vi "main.vi"() -> ()   [LabVIEW 2015]
uses:
  USB Template (LV 8.6)/Boiler/Controls/Boiler Controls.ctl
  USB Template (LV 8.6)/Boiler/Controls/Boiler Simulation Controls.ctl
  USB Template (LV 8.6)/Boiler/Controls/Boiler Status Indicators.ctl
  status.ctl
  boiler data.ctl
  log info.ctl
  timerstatus.ctl
panel:
  out "error out":errorcluster
  in  "stop":bool
  out "Boiler Status Indicators":T1 {"Time Count" format="%.2g"}
  in  "Boiler Simulation Controls":T2 {"Flame Sensor Value (%)" min=0.0 max=100.0 scale=0.0..100.0}
  in  "Boiler Controls":T3 {"Fuel Valve Position" min=0.0 max=100.0 scale=0.0..100.0 scale format="%.2f"}
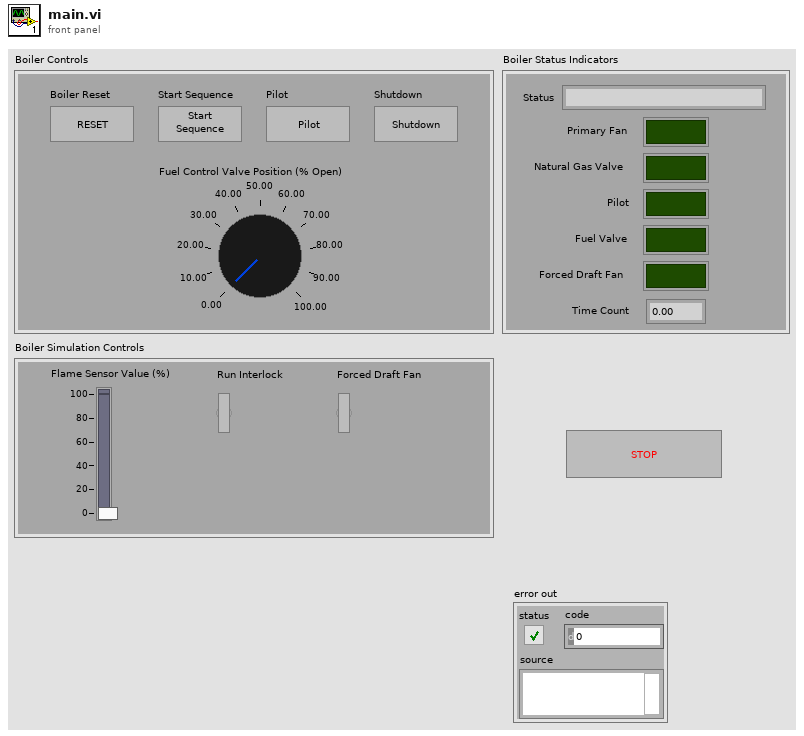
[diagram p1: front panel]
types:
  T1 = typedef "Boiler Status Indicators.ctl" = cluster{"Status":string, "Primary Fan":bool, "Natural Gas Valve":bool, "Pilot":bool, "Fuel Valve":bool, "Forced Draft Fan":bool, "Time Count":dbl}
  T2 = typedef "Boiler Simulation Controls.ctl" = cluster{"Flame Sensor Value (%)":dbl, "Run Interlock":bool, "Forced Draft Fan":bool}
  T3 = typedef "Boiler Controls.ctl" = cluster{"Boiler Reset":bool, "Start Sequence":bool, "Pilot":bool, "Shutdown":bool, "Fuel Valve Position":dbl}
  T4 = typedef "status.ctl" = enum16{"Shutdown", "Start", "Pilot on", "Error", "Running", "Purge", "Pilot proved", "PPCompleted", "Pre Purge", "Ready", "Exit", "Initialize"}
  T5 = typedef "log info.ctl" = cluster{"event":string, "data":string}
  T6 = typedef "timerstatus.ctl" = enum16{"Stop", "Start"}
  T7 = typedef "boiler data.ctl" = cluster{"Boiler Status Indicators":T1, "log path":path}
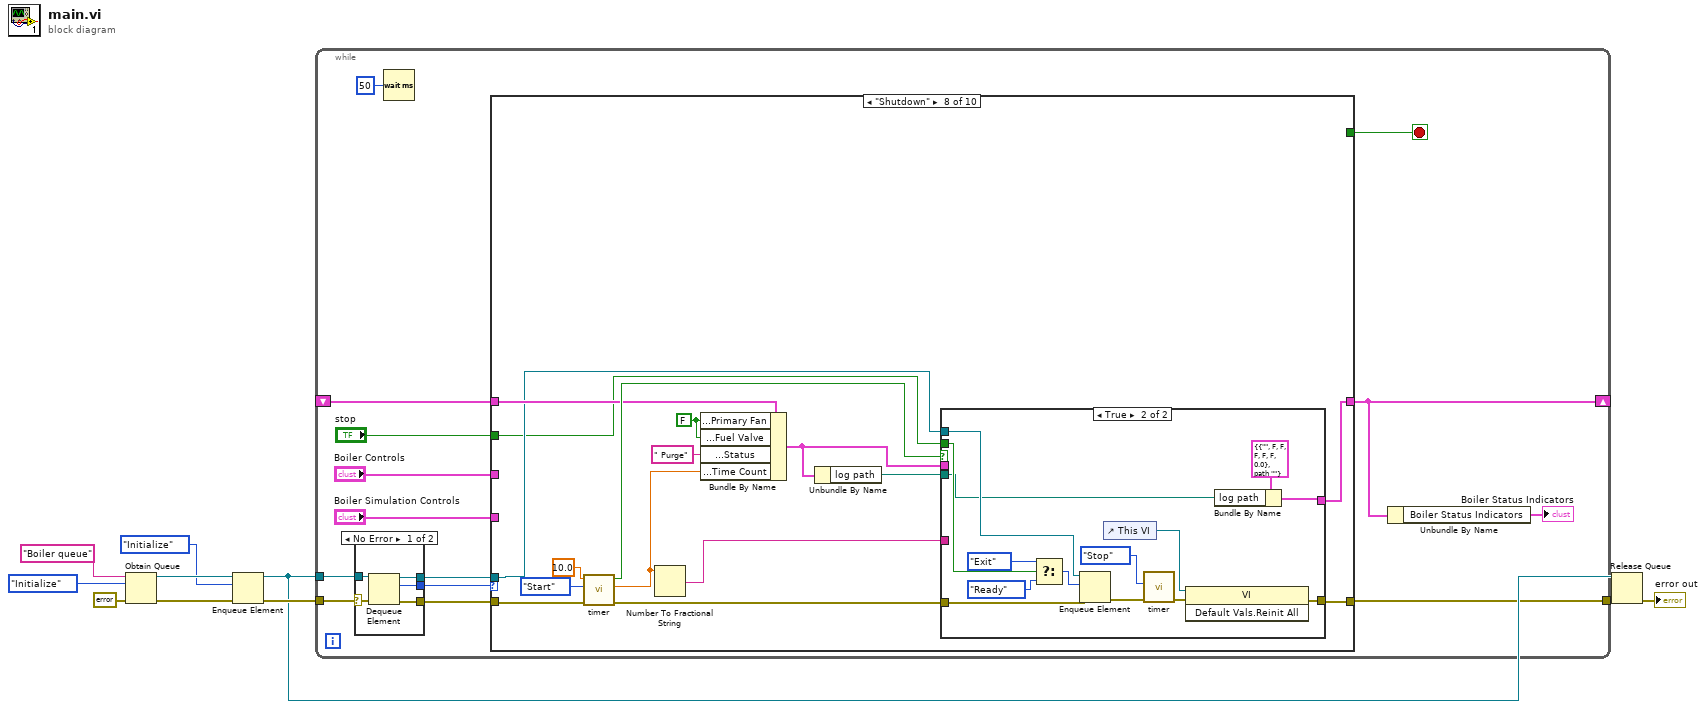
[diagram p0: block diagram]
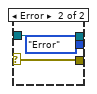
[diagram p2: hidden frame]
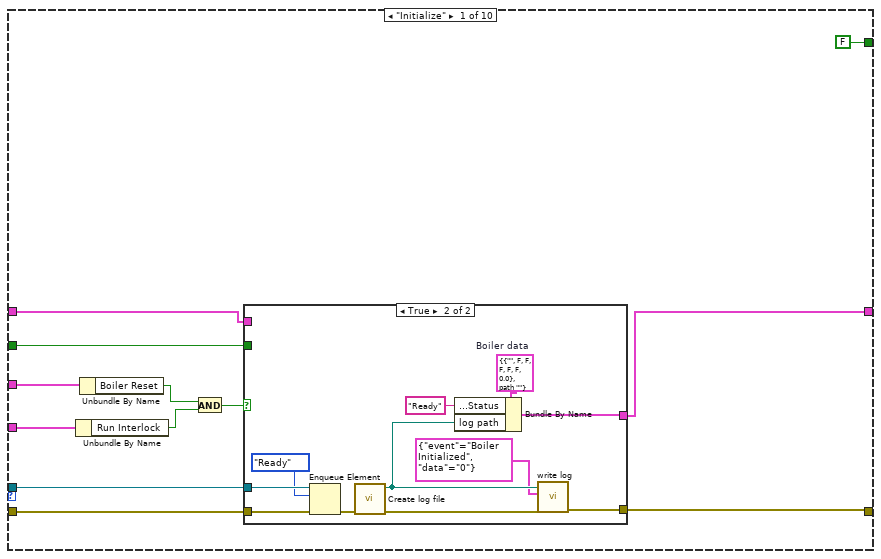
[diagram p3: hidden frame]
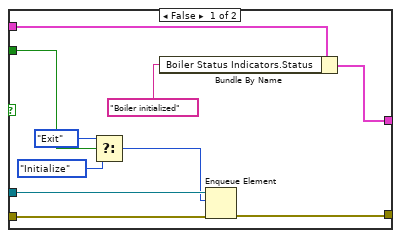
[diagram p4: hidden frame]
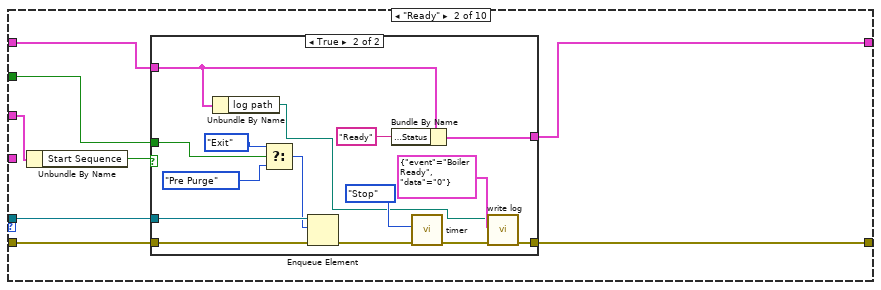
[diagram p5: hidden frame]
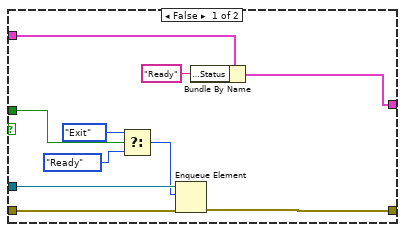
[diagram p6: hidden frame]
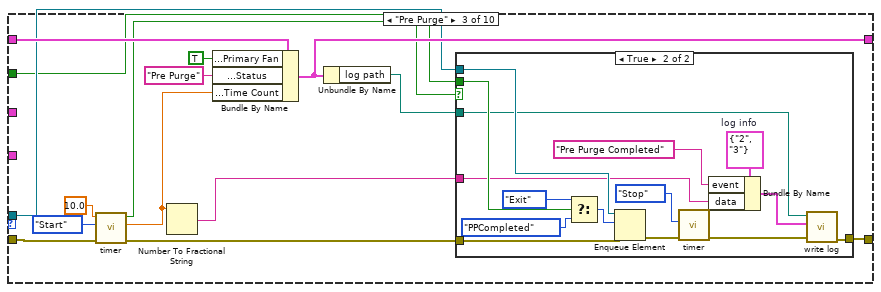
[diagram p7: hidden frame]
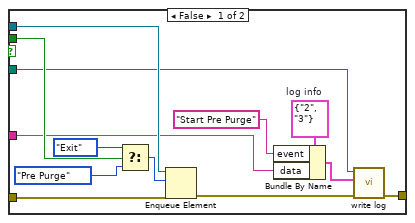
[diagram p8: hidden frame]
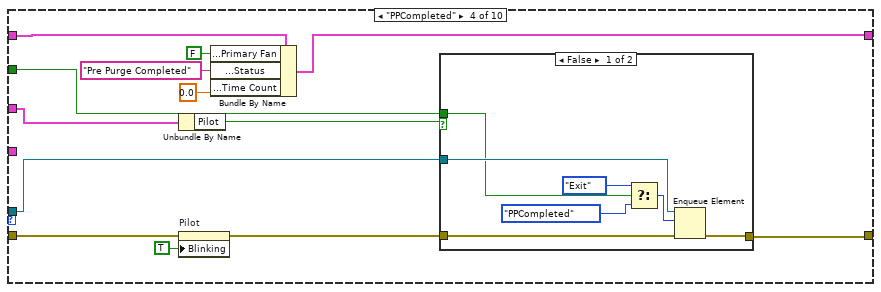
[diagram p9: hidden frame]
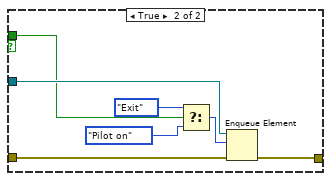
[diagram p10: hidden frame]
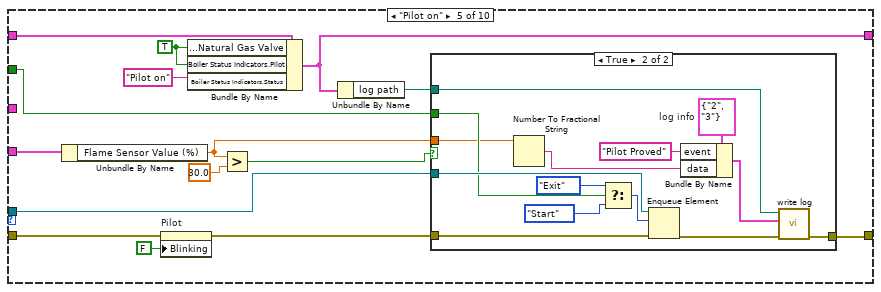
[diagram p11: hidden frame]
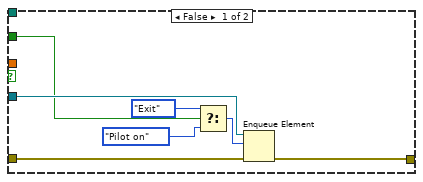
[diagram p12: hidden frame]
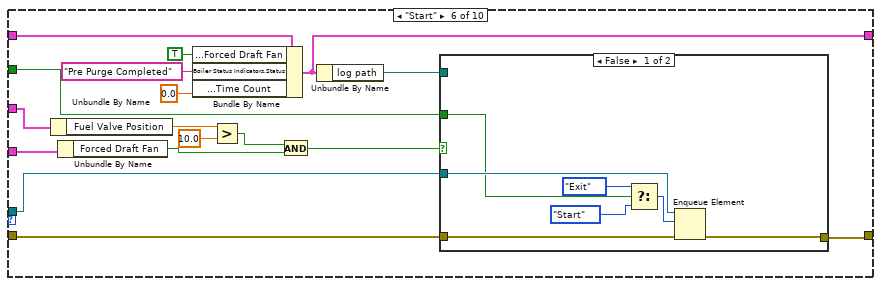
[diagram p13: hidden frame]
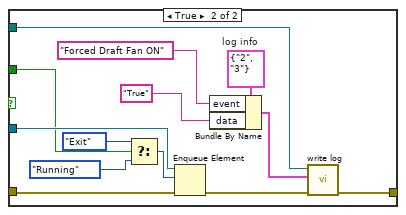
[diagram p14: hidden frame]
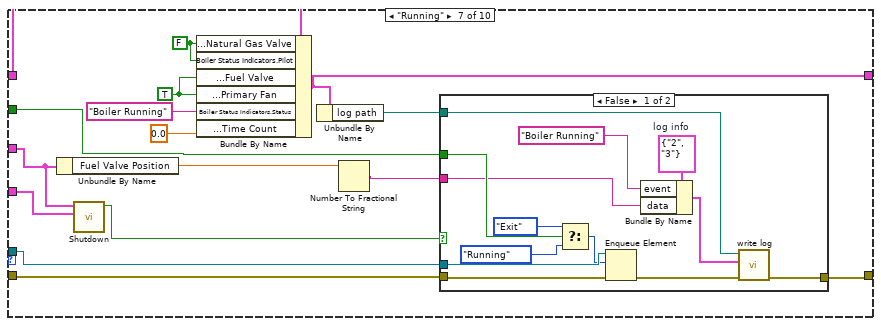
[diagram p15: hidden frame]
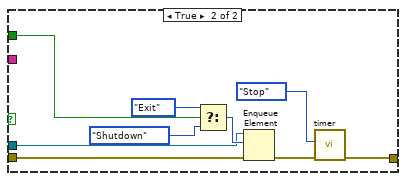
[diagram p16: hidden frame]
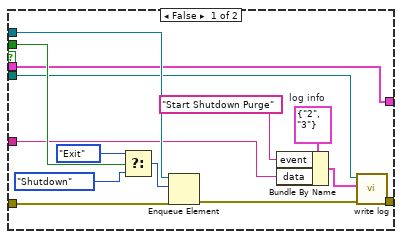
[diagram p17: hidden frame]
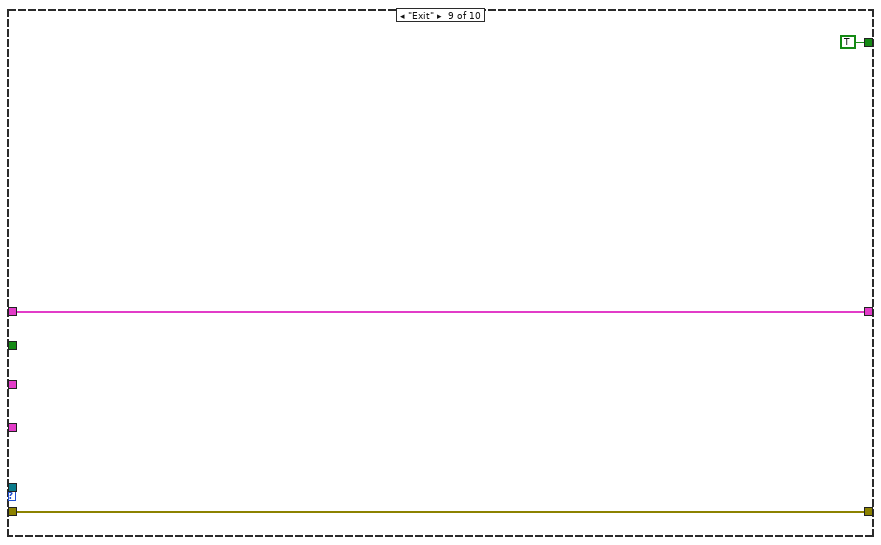
[diagram p18: hidden frame]
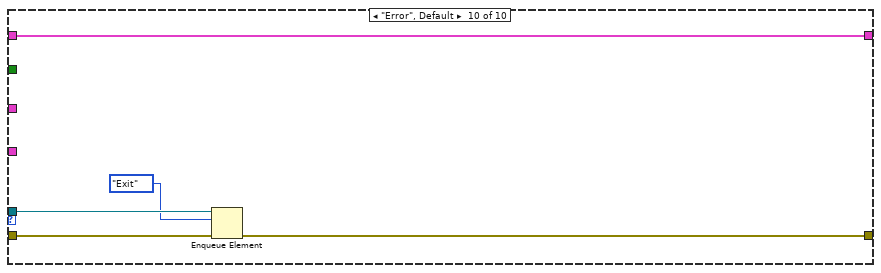
[diagram p19: hidden frame]
diagram:
  n1 = Obtain Queue(name (unnamed)="Boiler queue", element data type=status."Initialize" ("status"), error in (no error)=errorcluster {"status"=FALSE, "code"=0, "source"=""}) -> (queue out=w9:refnum<queue>, error out=w10:errorcluster)  [unwired: 2 in, 1 out]
  n2 = Enqueue Element(queue=w9, element=status."Initialize" ("status"), error in (no error)=w10) -> (queue out=w4:refnum<queue>, error out=w8:errorcluster)  [unwired: 1 in, 1 out]
  n3 = while {
    tunnel: w8 -> [w12]
    tunnel: w4 -> [w24]
    tunnel: [w20] -> w2
    shift-right: [w18] -> _
    shift-left: _ -> [w14]
    stop <- w19 stop-if-true
    n4 = case shown="No Error" w12 {
      selector: w12 -> [w25 w31]
      tunnel: w24 -> [w29 w32]
      tunnel: [w26 w31] -> w23
      tunnel: [w28 status."Error" ("status")] -> w22
      tunnel: [w27 w32] -> w21
      frame No Error {
        n5 = Dequeue Element(queue=w29, error in (no error)=w25) -> (queue out=w27:refnum<queue>, element=w28:T4, error out=w26:errorcluster)  [unwired: 1 in, 1 out]
      }
      frame Error {
      }
    }
    n6 = Wait (ms)(milliseconds to wait=u32 50) -> ()  [unwired: 1 out]
    n7 = case shown="\"Shutdown\"" w22 {
      tunnel: w23 -> [w42 w72 w112 w148 w182 w218 w254 w287 w325 w330]
      tunnel: w21 -> [w41 w71 w105 w142 w173 w217 w252 w284 _ w328]
      tunnel: [w43 w70 w100 w152 w180 w213 w253 w286 w325 w329] -> w20
      tunnel: [w39 w69 w106 w149 w170 w212 w250 w280 w324 w331] -> w18
      tunnel: [FALSE _ _ _ _ _ _ _ TRUE _] -> w19
      tunnel: "Boiler Simulation Controls" -> [w40 _ _ _ w176 w214 w244 _ _ _]
      tunnel: "Boiler Controls" -> [w38 w68 _ w145 _ w210 w243 _ _ _]
      tunnel: w14 -> [w34 w67 w110 w150 w179 w216 w251 w285 w324 w331]
      tunnel: "stop" -> [w33 w66 w103 w143 w172 w215 w245 w283 _ _]
      frame "Initialize" {
        n8 = Unbundle By Name(w40) -> ("Run Interlock"=w36:bool)
        n9 = Unbundle By Name(w38) -> ("Boiler Reset"=w37:bool)
        n10 = And(x=w37, y=w36) -> (x .and. y?=w35:bool)
        n11 = case shown="True" w35 {
          tunnel: [w46 w64] -> w39
          tunnel: [w53 w62] -> w43
          tunnel: w42 -> [w54 w59]
          tunnel: w41 -> [w52 w57]
          tunnel: w34 -> [w47 _]
          tunnel: w33 -> [w51 _]
          frame False {
            n12 = Select(t=status."Exit", s=w51, f=status."Initialize" ("element")) -> (s? t:f=w48:T4)
            n13 = Bundle By Name(cluster=w47, "Boiler Status Indicators.Status"="Boiler initialized" ("Status")) -> (w46:T7)
            n14 = Enqueue Element(queue=w52, element=w48, error in (no error)=w54) -> (error out=w53:errorcluster)  [unwired: 1 in, 2 out]
          }
          frame True {
            w65 = T7 {"Boiler Status Indicators"={"Status"="", "Primary Fan"=FALSE, "Natural Gas Valve"=FALSE, "Pilot"=FALSE, "Fuel Valve"=FALSE, "Forced Draft Fan"=FALSE, "Time Count"=0.0}, "log path"=path ""}  # Boiler data
            n15 = Enqueue Element(queue=w57, element=status."Ready", error in (no error)=w59) -> (error out=w58:errorcluster)  [unwired: 1 in, 2 out]
            n16 = call "Create log file.vi"("error in (no error)"=w58) -> ("error out"=w63:errorcluster, "log path"=w61:path)  [unwired: 9 in]
            n17 = Bundle By Name(cluster=w65, "Boiler Status Indicators.Status"="Ready", "log path"=w61) -> (w64:T7)
            n18 = call "write log.vi"("error in (no error)"=w63, "log info"=T5 {"event"="Boiler Initialized", "data"="0"}, "file"=w61) -> ("error out"=w62:errorcluster)  [unwired: 8 in]
          }
        }
      }
      frame "Ready" {
        n19 = Unbundle By Name(w68) -> ("Start Sequence"=w73:bool)
        n20 = case shown="True" w73 {
          tunnel: [w75 w98] -> w69
          tunnel: [w82 w97] -> w70
          tunnel: w72 -> [w83 w95]
          tunnel: w71 -> [w81 w94]
          tunnel: w67 -> [w76 w85]
          tunnel: w66 -> [w80 w89]
          frame False {
            n21 = Select(t=status."Exit", s=w80, f=status."Ready" ("element")) -> (s? t:f=w77:T4)
            n22 = Enqueue Element(queue=w81, element=w77, error in (no error)=w83) -> (error out=w82:errorcluster)  [unwired: 1 in, 2 out]
            n23 = Bundle By Name(cluster=w76, "Boiler Status Indicators.Status"="Ready") -> (w75:T7)
          }
          frame True {
            n24 = Unbundle By Name(w85) -> ("log path"=w84:path)
            n25 = Select(t=status."Exit", s=w89, f=status."Pre Purge" ("element")) -> (s? t:f=w86:T4)
            n26 = Enqueue Element(queue=w94, element=w86, error in (no error)=w95) -> (error out=w92:errorcluster)  [unwired: 1 in, 2 out]
            n27 = Bundle By Name(cluster=w85, "Boiler Status Indicators.Status"="Ready") -> (w98:T7)
            n28 = call "timer.vi"("error in (no error)"=w92, "timerstatus"=timerstatus."Stop") -> ("error out"=w91:errorcluster)  [unwired: 7 in, 2 out]
            n29 = call "write log.vi"("error in (no error)"=w91, "log info"=T5 {"event"="Boiler Ready", "data"="0"}, "file"=w84) -> ("error out"=w97:errorcluster)  [unwired: 8 in]
          }
        }
      }
      frame "Pre Purge" {
        n30 = call "timer.vi"("error in (no error)"=w112, "timerstatus"=timerstatus."Start", "limit"=10.0) -> ("error out"=w99:errorcluster, "elapsed"=w107:dbl, "out of limit"=w104:bool)  [unwired: 6 in]
        n31 = Number To Fractional String(number=w107) -> (F-format string=w101:string)  [unwired: 3 in]
        n32 = Bundle By Name(cluster=w110, "Boiler Status Indicators.Primary Fan"=TRUE, "Boiler Status Indicators.Status"="Pre Purge", "Boiler Status Indicators.Time Count"=w107) -> (w106:T7)
        n33 = Unbundle By Name(w106) -> ("log path"=w102:path)
        n34 = case shown="True" w104 {
          tunnel: w99 -> [w123 w134]
          tunnel: [w117 w132] -> w100
          tunnel: w105 -> [w122 w141]
          tunnel: w103 -> [w121 w140]
          tunnel: w102 -> [w115 w127]
          tunnel: w101 -> [w114 w129]
          frame False {
            w119 = T5 {"event"="2", "data"="3"}  # log info
            n35 = Select(t=status."Exit" ("status"), s=w121, f=status."Pre Purge" ("status")) -> (s? t:f=w125:T4)
            n36 = Enqueue Element(queue=w122, element=w125, error in (no error)=w123) -> (error out=w118:errorcluster)  [unwired: 1 in, 2 out]
            n37 = Bundle By Name(cluster=w119, "event"="Start Pre Purge", "data"=w114) -> (w120:T5)
            n38 = call "write log.vi"("error in (no error)"=w118, "log info"=w120, "file"=w115) -> ("error out"=w117:errorcluster)  [unwired: 8 in]
          }
          frame True {
            w130 = T5 {"event"="2", "data"="3"}  # log info
            n39 = Select(t=status."Exit" ("status"), s=w140, f=status."PPCompleted" ("status")) -> (s? t:f=w138:T4)
            n40 = Enqueue Element(queue=w141, element=w138, error in (no error)=w134) -> (error out=w136:errorcluster)  [unwired: 1 in, 2 out]
            n41 = call "timer.vi"("error in (no error)"=w136, "timerstatus"=timerstatus."Stop") -> ("error out"=w133:errorcluster)  [unwired: 7 in, 2 out]
            n42 = Bundle By Name(cluster=w130, "event"="Pre Purge Completed", "data"=w129) -> (w128:T5)
            n43 = call "write log.vi"("error in (no error)"=w133, "log info"=w128, "file"=w127) -> ("error out"=w132:errorcluster)  [unwired: 8 in]
          }
        }
      }
      frame "PPCompleted" {
        n44 = Unbundle By Name(w145) -> ("Pilot"=w144:bool)
        n45 = property on="Pilot" class="Bool (strict)"(error in=w148, "Blinking"=TRUE) -> (error out=w147:errorcluster)  [unwired: 1 in, 1 out]
        n46 = Bundle By Name(cluster=w150, "Boiler Status Indicators.Primary Fan"=FALSE, "Boiler Status Indicators.Status"="Pre Purge Completed", "Boiler Status Indicators.Time Count"=0.0 ("Time Count")) -> (w149:T7)
        n47 = case shown="False" w144 {
          tunnel: w147 -> [w158 w168]
          tunnel: [w157 w162] -> w152
          tunnel: w142 -> [w156 w167]
          tunnel: w143 -> [w155 w166]
          frame False {
            n48 = Select(t=status."Exit" ("status"), s=w155, f=status."PPCompleted" ("status")) -> (s? t:f=w160:T4)
            n49 = Enqueue Element(queue=w156, element=w160, error in (no error)=w158) -> (error out=w157:errorcluster)  [unwired: 1 in, 2 out]
          }
          frame True {
            n50 = Select(t=status."Exit" ("status"), s=w166, f=status."Pilot on" ("status")) -> (s? t:f=w164:T4)
            n51 = Enqueue Element(queue=w167, element=w164, error in (no error)=w168) -> (error out=w162:errorcluster)  [unwired: 1 in, 2 out]
          }
        }
      }
      frame "Pilot on" {
        w177 = TRUE ("Boiler Status Indicators.Primary Fan")
        n52 = Unbundle By Name(w176) -> ("Flame Sensor Value (%)"=w171:dbl)
        n53 = property on="Pilot" class="Bool (strict)"(error in=w182, "Blinking"=FALSE) -> (error out=w181:errorcluster)  [unwired: 1 in, 1 out]
        n54 = Bundle By Name(cluster=w179, "Boiler Status Indicators.Natural Gas Valve"=w177, "Boiler Status Indicators.Pilot"=w177, "Boiler Status Indicators.Status"="Pilot on") -> (w170:T7)
        n55 = Greater?(x=w171, y=30.0) -> (0:w174:bool)
        n56 = Unbundle By Name(w170) -> ("log path"=w169:path)
        n57 = case shown="True" w174 {
          tunnel: w181 -> [w187 w204]
          tunnel: [w186 w196] -> w180
          tunnel: w173 -> [w185 w203]
          tunnel: w172 -> [w184 w202]
          tunnel: w171 -> [_ w193]
          tunnel: w169 -> [_ w195]
          frame False {
            n58 = Select(t=status."Exit" ("status"), s=w184, f=status."Pilot on" ("status")) -> (s? t:f=w189:T4)
            n59 = Enqueue Element(queue=w185, element=w189, error in (no error)=w187) -> (error out=w186:errorcluster)  [unwired: 1 in, 2 out]
          }
          frame True {
            w198 = T5 {"event"="2", "data"="3"}  # log info
            n60 = Number To Fractional String(number=w193) -> (F-format string=w192:string)  [unwired: 3 in]
            n61 = Select(t=status."Exit" ("status"), s=w202, f=status."Start" ("status")) -> (s? t:f=w200:T4)
            n62 = Enqueue Element(queue=w203, element=w200, error in (no error)=w204) -> (error out=w197:errorcluster)  [unwired: 1 in, 2 out]
            n63 = Bundle By Name(cluster=w198, "event"="Pilot Proved", "data"=w192) -> (w191:T5)
            n64 = call "write log.vi"("error in (no error)"=w197, "log info"=w191, "file"=w195) -> ("error out"=w196:errorcluster)  [unwired: 8 in]
          }
        }
      }
      frame "Start" {
        n65 = Unbundle By Name(w210) -> ("Fuel Valve Position"=w209:dbl)
        n66 = Unbundle By Name(w214) -> ("Forced Draft Fan"=w206:bool)
        n67 = Bundle By Name(cluster=w216, "Boiler Status Indicators.Forced Draft Fan"=TRUE ("Boiler Status Indicators.Primary Fan"), "Boiler Status Indicators.Status"="Pre Purge Completed", "Boiler Status Indicators.Time Count"=0.0 ("Time Count")) -> (w212:T7)
        n68 = Greater?(x=w209, y=10.0) -> (0:w207:bool)
        n69 = And(x=w207, y=w206) -> (x .and. y?=w205:bool)
        n70 = Unbundle By Name(w212) -> ("log path"=w211:path)
        n71 = case shown="False" w205 {
          tunnel: w218 -> [w225 w241]
          tunnel: [w224 w233] -> w213
          tunnel: w217 -> [w223 w240]
          tunnel: w215 -> [w222 w239]
          tunnel: w211 -> [_ w231]
          frame False {
            n72 = Select(t=status."Exit" ("status"), s=w222, f=status."Start" ("status")) -> (s? t:f=w227:T4)
            n73 = Enqueue Element(queue=w223, element=w227, error in (no error)=w225) -> (error out=w224:errorcluster)  [unwired: 1 in, 2 out]
          }
          frame True {
            w235 = T5 {"event"="2", "data"="3"}  # log info
            n74 = Select(t=status."Exit" ("status"), s=w239, f=status."Running" ("status")) -> (s? t:f=w237:T4)
            n75 = Enqueue Element(queue=w240, element=w237, error in (no error)=w241) -> (error out=w234:errorcluster)  [unwired: 1 in, 2 out]
            n76 = Bundle By Name(cluster=w235, "event"="Forced Draft Fan ON", "data"="True") -> (w232:T5)
            n77 = call "write log.vi"("error in (no error)"=w234, "log info"=w232, "file"=w231) -> ("error out"=w233:errorcluster)  [unwired: 8 in]
          }
        }
      }
      frame "Running" {
        w248 = FALSE ("Boiler Status Indicators.Natural Gas Valve")
        w249 = TRUE ("Boiler Status Indicators.Primary Fan")
        n78 = Unbundle By Name(w243) -> ("Fuel Valve Position"=w247:dbl)
        n79 = call "Shutdown.vi"("Boiler Simulation Controls"=w244, "Boiler Controls"=w243) -> ("result"=w242:bool)  [unwired: 9 in]
        n80 = Bundle By Name(cluster=w251, "Boiler Status Indicators.Natural Gas Valve"=w248, "Boiler Status Indicators.Pilot"=w248, "Boiler Status Indicators.Fuel Valve"=w249, "Boiler Status Indicators.Primary Fan"=w249, "Boiler Status Indicators.Status"="Boiler Running", "Boiler Status Indicators.Time Count"=0.0 ("Time Count")) -> (w250:T7)
        n81 = Unbundle By Name(w250) -> ("log path"=w257:path)
        n82 = Number To Fractional String(number=w247) -> (F-format string=w246:string)  [unwired: 3 in]
        n83 = case shown="False" w242 {
          tunnel: w254 -> [w270 w276]
          tunnel: [w262 w272] -> w253
          tunnel: w252 -> [w269 w275]
          tunnel: w245 -> [w268 w274]
          tunnel: w257 -> [w260 _]
          tunnel: w246 -> [w258 _]
          frame False {
            w264 = T5 {"event"="2", "data"="3"}  # log info
            n84 = Select(t=status."Exit" ("status"), s=w268, f=status."Running" ("status")) -> (s? t:f=w266:T4)
            n85 = Enqueue Element(queue=w269, element=w266, error in (no error)=w270) -> (error out=w263:errorcluster)  [unwired: 1 in, 2 out]
            n86 = Bundle By Name(cluster=w264, "event"="Boiler Running", "data"=w258) -> (w261:T5)
            n87 = call "write log.vi"("error in (no error)"=w263, "log info"=w261, "file"=w260) -> ("error out"=w262:errorcluster)  [unwired: 8 in]
          }
          frame True {
            n88 = Select(t=status."Exit" ("status"), s=w274, f=status."Shutdown" ("status")) -> (s? t:f=w278:T4)
            n89 = Enqueue Element(queue=w275, element=w278, error in (no error)=w276) -> (error out=w273:errorcluster)  [unwired: 1 in, 2 out]
            n90 = call "timer.vi"("error in (no error)"=w273, "timerstatus"=timerstatus."Stop") -> ("error out"=w272:errorcluster)  [unwired: 7 in, 2 out]
          }
        }
      }
      frame "Shutdown" {
        w282 = FALSE ("Boiler Status Indicators.Primary Fan")
        n91 = call "timer.vi"("error in (no error)"=w287, "timerstatus"=timerstatus."Start", "limit"=10.0) -> ("error out"=w295:errorcluster, "elapsed"=w291:dbl, "out of limit"=w292:bool)  [unwired: 6 in]
        n92 = Number To Fractional String(number=w291) -> (F-format string=w294:string)  [unwired: 3 in]
        n93 = Bundle By Name(cluster=w285, "Boiler Status Indicators.Primary Fan"=w282, "Boiler Status Indicators.Fuel Valve"=w282, "Boiler Status Indicators.Status"=" Purge", "Boiler Status Indicators.Time Count"=w291) -> (w281:T7)
        n94 = Unbundle By Name(w281) -> ("log path"=w293:path)
        n95 = case shown="True" w292 {
          tunnel: w295 -> [w306 w316]
          tunnel: [w300 w311] -> w286
          tunnel: w284 -> [w305 w323]
          tunnel: w283 -> [w304 w322]
          tunnel: w293 -> [w298 w314]
          tunnel: w294 -> [w297 _]
          tunnel: w281 -> [w296 _]
          tunnel: [w296 w313] -> w280
          frame False {
            w302 = T5 {"event"="2", "data"="3"}  # log info
            n96 = Select(t=status."Exit" ("status"), s=w304, f=status."Shutdown" ("status")) -> (s? t:f=w308:T4)
            n97 = Enqueue Element(queue=w305, element=w308, error in (no error)=w306) -> (error out=w301:errorcluster)  [unwired: 1 in, 2 out]
            n98 = Bundle By Name(cluster=w302, "event"="Start Shutdown Purge", "data"=w297) -> (w303:T5)
            n99 = call "write log.vi"("error in (no error)"=w301, "log info"=w303, "file"=w298) -> ("error out"=w300:errorcluster)  [unwired: 8 in]
          }
          frame True {
            n100 = Select(t=status."Exit" ("status"), s=w322, f=status."Ready" ("status")) -> (s? t:f=w320:T4)
            n101 = Enqueue Element(queue=w323, element=w320, error in (no error)=w316) -> (error out=w318:errorcluster)  [unwired: 1 in, 2 out]
            n102 = control-ref of="This VI"() -> (w310:refnum<vi>)
            n103 = call "timer.vi"("error in (no error)"=w318, "timerstatus"=timerstatus."Stop") -> ("error out"=w312:errorcluster)  [unwired: 7 in, 2 out]
            n104 = invoke class="VI" method="Default Vals.Reinit All"(reference=w310, error in=w312) -> (error out=w311:errorcluster)  [unwired: 1 in, 2 out]
            n105 = Bundle By Name(cluster=T7 {"Boiler Status Indicators"={"Status"="", "Primary Fan"=FALSE, "Natural Gas Valve"=FALSE, "Pilot"=FALSE, "Fuel Valve"=FALSE, "Forced Draft Fan"=FALSE, "Time Count"=0.0}, "log path"=path ""} ("Boiler data"), "log path"=w314) -> (w313:T7)
          }
        }
      }
      frame "Exit" {
      }
      frame "Error", Default {
        n106 = Enqueue Element(queue=w328, element=status."Exit" ("status"), error in (no error)=w330) -> (error out=w329:errorcluster)  [unwired: 1 in, 2 out]
      }
    }
    n107 = Unbundle By Name(w18) -> ("Boiler Status Indicators"=→"Boiler Status Indicators":T1)
  }
  n108 = Release Queue(queue=w4, error in (no error)=w2) -> (error out=→"error out":errorcluster)  [unwired: 1 in, 2 out]
